vi "Stabilization Naked Sphere FGV.vi"(10 "Control":enum16{"reset", "add"}(ring), 11 "Stabilization Value In":dbl format="%#_13g") -> (3 "Stabilization Array Out":dbl[](array[numeric]))   [LabVIEW 2014, in "Timing and Stabilization.lvlib"]
uses:
  Timing and Stabilization.lvlib
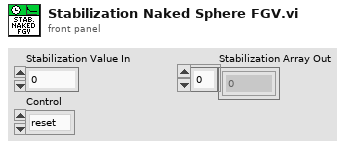
[diagram p1: front panel]
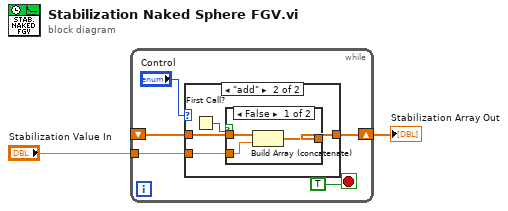
[diagram p0: block diagram]
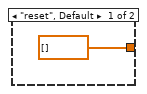
[diagram p2: hidden frame]
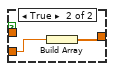
[diagram p3: hidden frame]
diagram:
  n1 = while {
    tunnel: "Stabilization Value In" -> [w7]
    shift-right: [w5] -> w1
    shift-left: _ -> [w6]
    stop <- TRUE stop-if-true
    n2 = case shown="\"add\"" "Control" {
      tunnel: w7 -> [_ w12]
      tunnel: w6 -> [_ w11]
      tunnel: [dbl[] [] w10] -> w5
      frame "reset", Default {
      }
      frame "add" {
        n3 = First Call?() -> (First Call?: T/F=w9:bool)
        n4 = case shown="False" w9 {
          tunnel: w12 -> [w15 w17]
          tunnel: w11 -> [w14 _]
          tunnel: [w13 w16] -> w10
          frame False {
            n5 = Build Array (concatenate)(w14, w15) -> (w13:dbl[])
          }
          frame True {
            n6 = Build Array(w17) -> (w16:dbl[])
          }
        }
      }
    }
  }
  "Stabilization Array Out" <- w1
